vi "iptest.vi"() -> ()   [LabVIEW 2025]
panel:
  out "Array":string[](array[string])
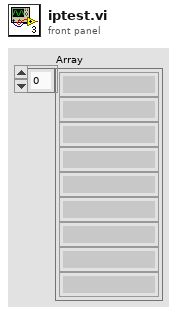
[diagram p1: front panel]
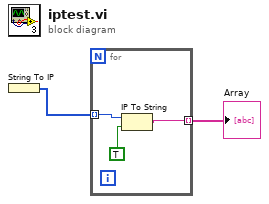
[diagram p0: block diagram]
diagram:
  n1 = String To IP() -> (0:w2:u32[])  [unwired: 1 in]
  n2 = for {
    tunnel: w2 -> [w5] mode=indexing
    tunnel: [w3] -> w1 mode=indexing
    n3 = IP To String(1:TRUE ("dot notation? (F)"), 2:w5) -> (0:w3:string)
  }
  "Array" <- w1
